vi "layout.vi"(0 "reference":refnum<class "ActorNode.lvclass">, 1 "graph":refnum<class "Graph.lvclass">, 2 "graphics":refnum<class "Graphics.lvclass">, 3 "grid":refnum<class "Grid.lvclass">, 5 "error in (no error)":errorcluster) -> (14 "reference out":refnum<class "ActorNode.lvclass">, 19 "error out":errorcluster)   [LabVIEW 2014, in "ActorNode.lvclass"]
uses:
  <resource>/Framework/Providers/Open_GDS/UML/ActorNode_class/ActorNode.lvclass
  <resource>/Framework/Providers/Open_GDS/UML/Graph_class/Graph.lvclass
  <resource>/Framework/Providers/Open_GDS/UML/Graphics_class/Graphics.lvclass
  <resource>/Framework/Providers/Open_GDS/UML/Grid_class/Grid.lvclass
  <resource>/Framework/Providers/Open_GDS/UML/MultiLineString_class/MultiLineString.lvclass
  <resource>/Framework/Providers/Open_GDS/UML/RectangularNode_class/RectangularNode.lvclass
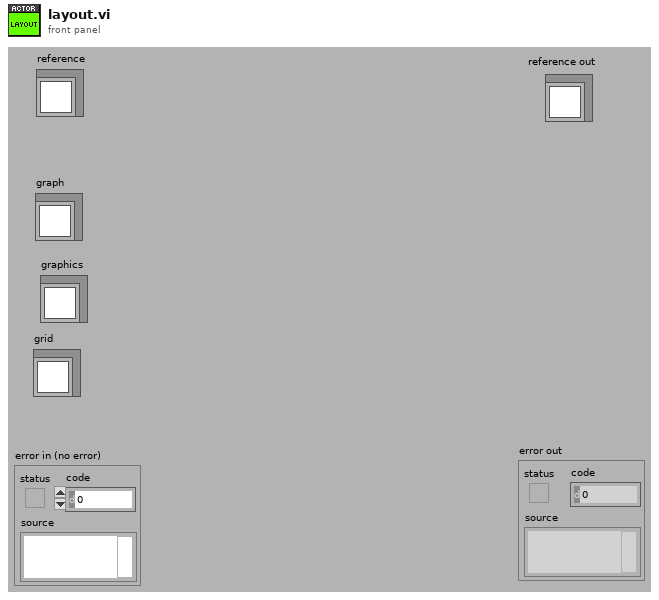
[diagram p1: front panel]
types:
  T1 = typedef "ActorNode.lvclass/ObjectAttributes.ctl" = cluster{"name":refnum<class "MultiLineString.lvclass">, "DEFAULT_WIDTH":i32, "DEFAULT_HEIGHT":i32, "DEFAULT_GAP":i32}
  T2 = typedef "RectangularNode.lvclass/ObjectAttributes.ctl" = cluster{"bounds":T3}
  T3 = typedef "Rectangle Rectangle2D.ctl" = cluster{"x":dbl, "y":dbl, "width":dbl, "height":dbl}
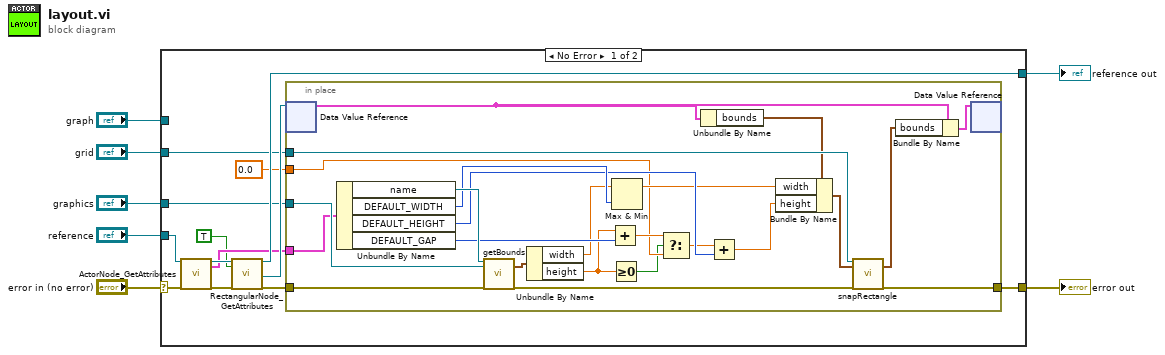
[diagram p0: block diagram]
diagram:
  n1 = case shown="No Error" "error in (no error)" {
    selector: "error in (no error)" -> [w18 w45]
    tunnel: "reference" -> [w20 w46]
    tunnel: [w11 w45] -> w6
    tunnel: [w19 w46] -> w5
    tunnel: "graph" -> [_ _]
    tunnel: "graphics" -> [w14 _]
    tunnel: "grid" -> [w12 _]
    frame No Error {
      n2 = call <resource>:"ActorNode_GetAttributes.vi"("reference in"=w20, "error in (no error)"=w18) -> ("reference out"=w17:refnum<class "ActorNode.lvclass">, "Data"=w9:T1, "error out"=w16:errorcluster)  [unwired: 14 in, 1 out]
      n3 = call <resource>:"RectangularNode_GetAttributes.vi"("reference in"=w17, "OnlyGetDvrReference(False)"=TRUE, "error in (no error)"=w16) -> ("reference out"=w19:refnum<class "ActorNode.lvclass">, "DataRef"=w15:refnum<data-value>, "error out"=w13:errorcluster)  [unwired: 13 in, 1 out]
      n4 = in-place {
        in-place-border: w14 -> [w40]
        in-place-border: w13 -> [w39]
        in-place-border: w12 -> [w30]
        in-place-border: [w27] -> w11
        in-place-border: 0.0 ("f") -> [w25]
        in-place-border: w9 -> [w21]
        n5 = in-place-dvr #1(w15) -> (w23:T2)  [unwired: 1 out]
        n6 = Unbundle By Name(w21) -> ("name"=w44:refnum<class "MultiLineString.lvclass">, "DEFAULT_WIDTH"=w43:i32, "DEFAULT_HEIGHT"=w42:i32, "DEFAULT_GAP"=w41:i32)
        n7 = call-dynamic "getBounds.vi"("reference"=w44, "graphics"=w40, "error in (no error)"=w39) -> ("bounds"=w38:T3, "error out"=w37:errorcluster)  [unwired: 15 out]
        n8 = Unbundle By Name(w38) -> ("width"=w36:dbl, "height"=w32:dbl)
        n9 = Add(x=w32, y=w41) -> (x+y=w31:dbl)
        n10 = Greater Or Equal To 0?(x=w32) -> (x >= 0?=w24:bool)
        n11 = Max & Min(x=w36, y=w43) -> (max(x,y)=w35:dbl)  [unwired: 1 out]
        n12 = Select(t=w31, s=w24, f=w25) -> (s? t:f=w34:dbl)
        n13 = Unbundle By Name(w23) -> ("bounds"=w26:T3)
        n14 = Add(x=w34, y=w42) -> (x+y=w33:dbl)
        n15 = Bundle By Name(cluster=w26, "width"=w35, "height"=w33) -> (w29:T3)
        n16 = call <resource>:"snapRectangle.vi"("reference"=w30, "bounds"=w29, "error in (no error)"=w37) -> ("boundsOut"=w28:T3, "error out"=w27:errorcluster)  [unwired: 15 out]
        n17 = Bundle By Name(cluster=w23, "bounds"=w28) -> (w22:T2)
        n18 = in-place-dvr #1(w22) -> ()  [unwired: 2 out]
      }
    }
    frame Error {
    }
  }
  "reference out" <- w5
  "error out" <- w6
